vi "Decimate2DArray.vi"(3 "Décimer y":i32, 4 "Décimer x":i32, 5 "Image Pixels (Float)":sgl[][](array[numeric])) -> (2 "Tableau":sgl[][](array[numeric]))   [LabVIEW 2014]
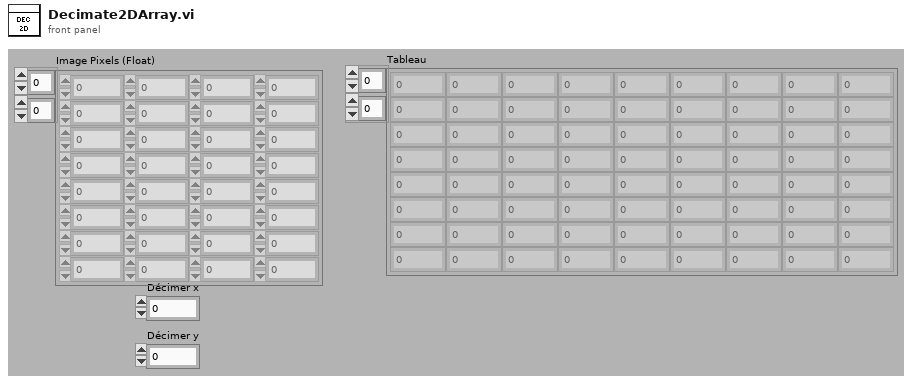
[diagram p1: front panel]
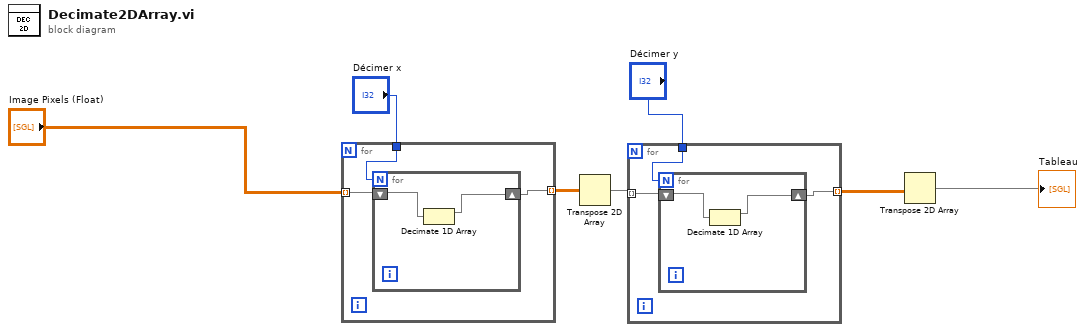
[diagram p0: block diagram]
diagram:
  n1 = for {
    tunnel: [w8] -> w7 mode=indexing
    tunnel: "Image Pixels (Float)" -> [w10] mode=indexing
    tunnel: "Décimer x" -> [w9]
    n2 = for {
      N: w9 -> [_]
      shift-right: [w11] -> w8
      shift-left: w10 -> [w12]
      n3 = Decimate 1D Array(w12) -> (w11:sgl[])  [unwired: 1 out]
    }
  }
  n4 = Transpose 2D Array(2D array=w7) -> (transposed array=w5:sgl[][])
  n5 = for {
    tunnel: [w13] -> w2 mode=indexing
    tunnel: w5 -> [w15] mode=indexing
    tunnel: "Décimer y" -> [w14]
    n6 = for {
      N: w14 -> [_]
      shift-right: [w16] -> w13
      shift-left: w15 -> [w17]
      n7 = Decimate 1D Array(w17) -> (w16:sgl[])  [unwired: 1 out]
    }
  }
  n8 = Transpose 2D Array(2D array=w2) -> (transposed array=→"Tableau":sgl[][])
